vi "Write Multiple.vi"(8 "error in (no error)":errorcluster, 9 "Values":variant[](array[variant]), 10 "Names":string[](array[string]), 11 "TwinCAT ADS in":refnum<class "TwinCAT ADS.lvclass">) -> (0 "error out":errorcluster, 3 "TwinCAT ADS out":refnum<class "TwinCAT ADS.lvclass">)   [LabVIEW 2018, in "TwinCAT ADS.lvclass"]
uses:
  TwinCAT ADS.lvclass
  TwinCAT.Ads
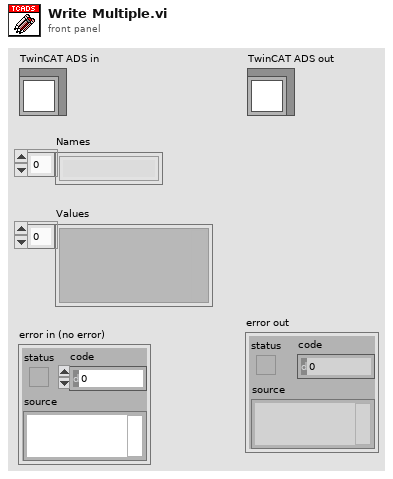
[diagram p1: front panel]
types:
  T1 = typedef "TwinCAT ADS.lvclass/Symbol Information.ctl" = cluster{"Name":string, "Short Name":string, "Size":i32, "Type Category":i32, "Type Name":string, "Type ID":i32, "Index Group":i64, "Index Offset":i64, "Child Count":i32, "Has Rpc Methods?":bool, "Comment":string}
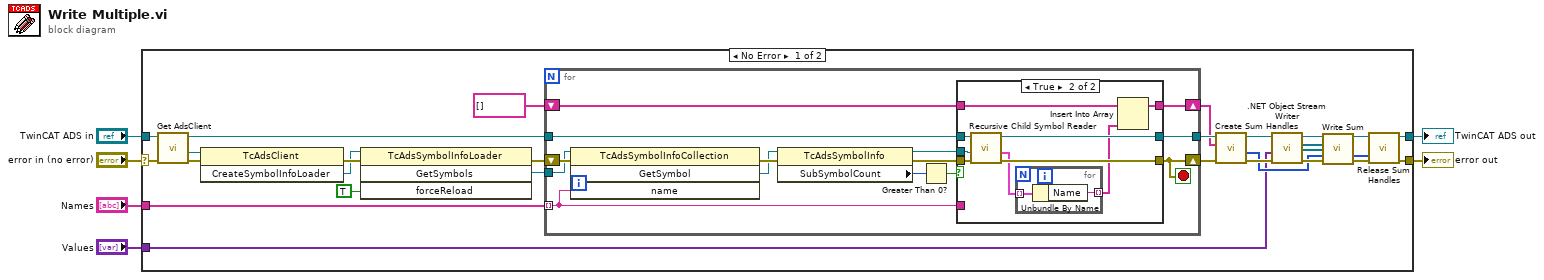
[diagram p0: block diagram]
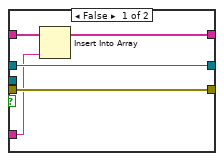
[diagram p2: hidden frame]
diagram:
  n1 = case shown="No Error" "error in (no error)" {
    selector: "error in (no error)" -> [w32 w66]
    tunnel: [w9 w66] -> w5
    tunnel: [w10 w65] -> w3
    tunnel: "TwinCAT ADS in" -> [w31 w65]
    tunnel: "Names" -> [w27 _]
    tunnel: "Values" -> [w7 _]
    frame No Error {
      n2 = call-dynamic "Get AdsClient.vi"("error in (no error)"=w32, "TwinCAT ADS in"=w31) -> ("error out"=w30:errorcluster, ".NET TcAdsClient refnum"=w29:refnum<k24>, "TwinCAT ADS out"=w25:refnum<class "TwinCAT ADS.lvclass">)  [unwired: 7 in]
      n3 = invoke class="TcAdsClient" method="CreateSymbolInfoLoader"(reference=w29, error in=w30) -> (error out=w34:errorcluster, "CreateSymbolInfoLoader"=w8:refnum<k24>)  [unwired: 1 in, 1 out]
      n4 = invoke class="TcAdsSymbolInfoLoader" method="GetSymbols"(reference=w8, error in=w34, "forceReload"=TRUE) -> (error out=w28:errorcluster, "GetSymbols"=w26:refnum<k24>)  [unwired: 1 in, 2 out]
      n5 = for {
        tunnel: w27 -> [w35] mode=indexing
        tunnel: w26 -> [w47]
        shift-right: [w38] -> w21
        shift-left: string[] [] -> [w39]
        shift-right: [w37] -> w23
        shift-left: w28 -> [w48]
        tunnel: w25 -> [w40]
        tunnel: [w36] -> w22
        stop <- w37 stop-if-true
        n6 = invoke class="TcAdsSymbolInfoCollection" method="GetSymbol"(reference=w47, error in=w48, "name"=w35) -> (error out=w46:errorcluster, "GetSymbol"=w45:refnum<k24>)  [unwired: 1 in, 2 out]
        n7 = property class="TcAdsSymbolInfo"(reference=w45, error in=w46) -> (reference out=w43:refnum<k24>, error out=w41:errorcluster, "SubSymbolCount"=w42:i32)
        n8 = Greater Than 0?(x=w42) -> (x > 0?=w44:bool)
        n9 = case shown="True" w44 {
          tunnel: w43 -> [_ w60]
          tunnel: w41 -> [w51 w62]
          tunnel: [w51 w56] -> w37
          tunnel: [w52 w58] -> w38
          tunnel: w40 -> [w50 w61]
          tunnel: [w50 w57] -> w36
          tunnel: w39 -> [w53 w59]
          tunnel: w35 -> [w49 _]
          frame False {
            n10 = Insert Into Array(array=w53, new element=w49) -> (w52:string[])  [unwired: 1 in]
          }
          frame True {
            n11 = call "Recursive Child Symbol Reader.vi"("error in (no error)"=w62, ".NET TcAdsSymbolInfo"=w60, "TwinCAT ADS in"=w61) -> ("error out"=w56:errorcluster, "Symbols Information"=w55:T1[], "TwinCAT ADS out"=w57:refnum<class "TwinCAT ADS.lvclass">)  [unwired: 6 in]
            n12 = for {
              tunnel: w55 -> [w64] mode=indexing
              tunnel: [w63] -> w54 mode=indexing
              n13 = Unbundle By Name(w64) -> ("Name"=w63:string)
            }
            n14 = Insert Into Array(array=w59, new element=w54) -> (w58:string[])  [unwired: 1 in]
          }
        }
      }
      n15 = call-dynamic "Create Sum Handles.vi"("error in (no error)"=w23, "Names"=w21, "TwinCAT ADS in"=w22) -> ("error out"=w19:errorcluster, "Handles"=w16:u32[], "TwinCAT ADS out"=w20:refnum<class "TwinCAT ADS.lvclass">)  [unwired: 6 in]
      n16 = call ".NET Object Stream Writer.vi"("error in (no error)"=w19, "G Object"=w7, "TwinCAT ADS in"=w20) -> ("error out"=w18:errorcluster, ".NET Object Stream"=w15:refnum<k24>[], ".NET Type Stream"=w14:refnum<k24>[], "TwinCAT ADS out"=w17:refnum<class "TwinCAT ADS.lvclass">)  [unwired: 5 in]
      n17 = call-dynamic "Write Sum.vi"("TwinCAT ADS in"=w17, ".NET Type Stream"=w14, ".NET Object Stream"=w15, "Handles"=w16, "error in (no error)"=w18) -> ("TwinCAT ADS out"=w12:refnum<class "TwinCAT ADS.lvclass">, "Handles"=w11:u32[], "error out"=w13:errorcluster)  [unwired: 8 in]
      n18 = call-dynamic "Release Sum Handles.vi"("error in (no error)"=w13, "Handles"=w11, "TwinCAT ADS in"=w12) -> ("error out"=w9:errorcluster, "TwinCAT ADS out"=w10:refnum<class "TwinCAT ADS.lvclass">)  [unwired: 7 in]
    }
    frame Error {
    }
  }
  "error out" <- w5
  "TwinCAT ADS out" <- w3
